vi "Quellenregler.vi"(0 "Regelung Quelle":bool, 2 "TI 38 IW °C":dbl, 3 "LEDs":bool[](array[boolean]), 5 "TI 38 SW °C":dbl=40.0 min=30.0 max=60.0) -> (6 "Ja!":bool, 7 "Kerzen von Regler":bool[](array[boolean]))   [LabVIEW 2015]
panel:
  in  "TI 37 IW °C":dbl
  in  "SP6":dbl=0.3
  in  "SP5":dbl=0.25
  out "e1":dbl
  in  "SP2":dbl=0.1
  in  "SP4":dbl=0.2
  in  "SP1":dbl=0.05
  in  "SP3":dbl=0.15
  # "Regelparameter"
  # "Kerzen manuell zuschalten?"
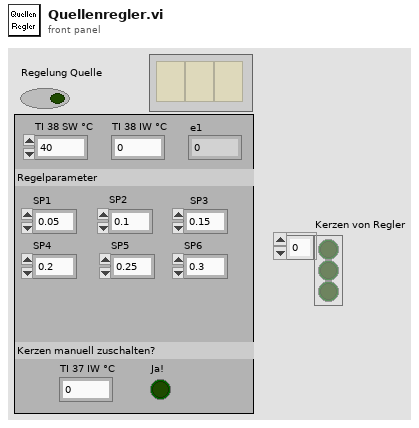
[diagram p1: front panel]
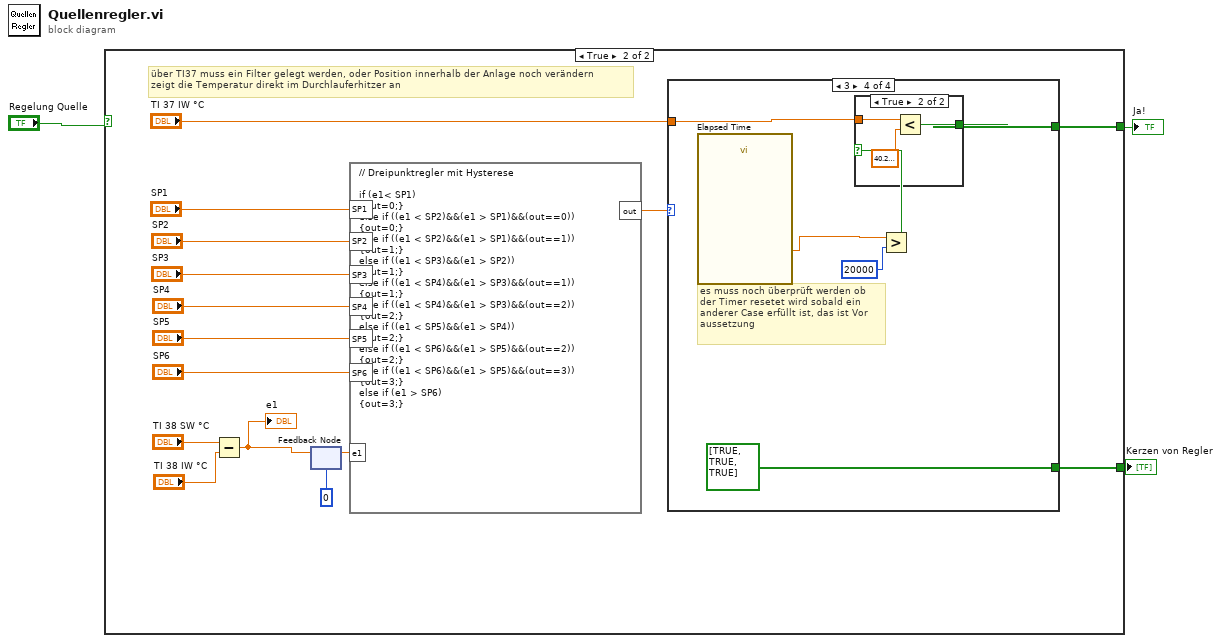
[diagram p0: block diagram]
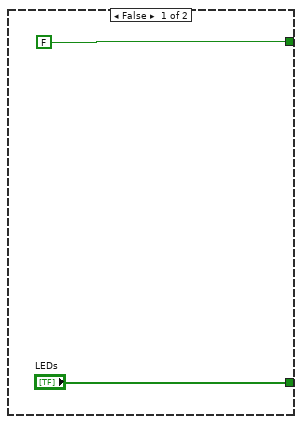
[diagram p2: hidden frame]
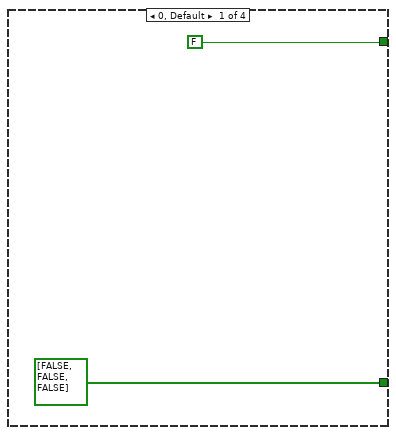
[diagram p3: hidden frame]
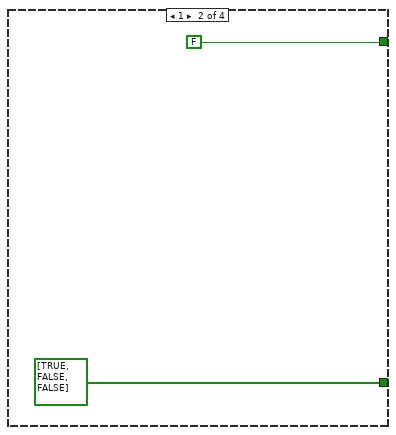
[diagram p4: hidden frame]
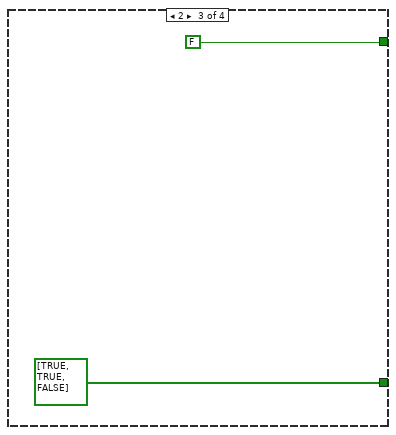
[diagram p5: hidden frame]
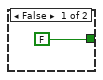
[diagram p6: hidden frame]
diagram:
  n1 = case shown="True" "Regelung Quelle" {
    tunnel: ["LEDs" w9] -> w2
    tunnel: [FALSE w7] -> w1
    frame False {
    }
    frame True {
      # "über TI37 muss ein Filter gelegt werden, oder Position innerhalb der Anlage noch verändern\nzeigt die Temperatur direkt im Durchlauferhitzer an"
      n2 = Subtract(x="TI 38 SW °C", y="TI 38 IW °C") -> (x-y=w6:dbl)
      "e1" <- w6
      n3 = feedback-in #1(w6) -> ()
      n4 = feedback #1(0) -> (w16:dbl)
      n5 = formula code="// Dreipunktregler mit Hysterese\n\nif (e1< SP1)\n{out=0;}\nelse if ((e1 < SP2)&&(e1 > SP1)&&(out==0))\n{out=0;}\nelse if ((e1 < SP2)&&(e1 > SP1)&&(out==1))\n{out=1;}\nelse if ((e1 < SP3)&&(e1 > SP2))\n{out=1;}\nelse if ((e1 < SP4)&&(e1 > SP3)&&(out==1))\n{out=1;}\nelse if ((e1 < SP4)&&(e1 > SP3)&&(out==2))\n{out=2;}\nelse if ((e1 < SP5)&&(e1 > SP4))\n{out=2;}\nelse if ((e1 < SP6)&&(e1 > SP5)&&(out==2))\n{out=2;}\nelse if ((e1 < SP6)&&(e1 > SP5)&&(out==3))\n{out=3;}\nelse if (e1 > SP6)\n{out=3;}"("e1"=w16, "SP1"="SP1", "SP3"="SP3", "SP4"="SP4", "SP2"="SP2", "SP5"="SP5", "SP6"="SP6") -> ("out"=w10:dbl)
      n6 = case shown="3" w10 {
        tunnel: [bool[] [FALSE, FALSE, FALSE] bool[] [TRUE, FALSE, FALSE] bool[] [TRUE, TRUE, FALSE] bool[] [TRUE, TRUE, TRUE]] -> w9
        tunnel: "TI 37 IW °C" -> [_ _ _ w31]
        tunnel: [FALSE FALSE FALSE w28] -> w7
        frame 0, Default {
        }
        frame 1 {
        }
        frame 2 {
        }
        frame 3 {
          # "es muss noch überprüft werden ob\nder Timer resetet wird sobald ein\nanderer Case erfüllt ist, das ist Vor\naussetzung"
          n7 = call "Elapsed Time"() -> ("Elapsed Time (s)"=w27:dbl)  [unwired: 12 in, 7 out]
          n8 = Greater?(x=w27, y=20000) -> (0:w29:bool)
          n9 = case shown="True" w29 {
            tunnel: w31 -> [_ w35]
            tunnel: [FALSE w34] -> w28
            frame False {
            }
            frame True {
              n10 = Less?(x=w35, y=sgl 40.2) -> (x < y?=w34:bool)
            }
          }
        }
      }
    }
  }
  "Kerzen von Regler" <- w2
  "Ja!" <- w1
